vi "Set All Elements.vi"(8 "error in":errorcluster, 10 "Channel Node":refnum<k20>, 11 "Channel Ref in":refnum<data-value>) -> (0 "error out":errorcluster, 3 "Channel Ref out":refnum<data-value>)   [LabVIEW 2024, in "Config File Parser.lvlib" / "Channel.lvclass"]
uses:
  Channel.lvclass
  Channel.lvclass/Channel.ctl
  <vilib>/xml/Close Reference(Node).vi
  Config File Parser.lvlib
  <resource>/objmgr/DOMUserDefRef.rc
  <vilib>/xml/NI_XML.lvlib
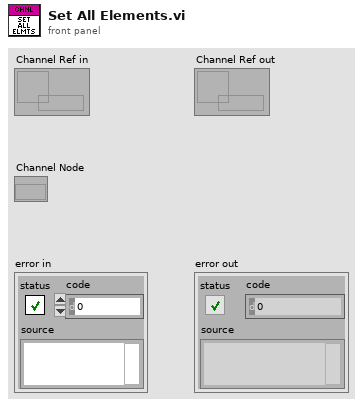
[diagram p1: front panel]
types:
  T1 = cluster{"Key":string, "IsError":bool, "Code":u32, "Message":string}[]
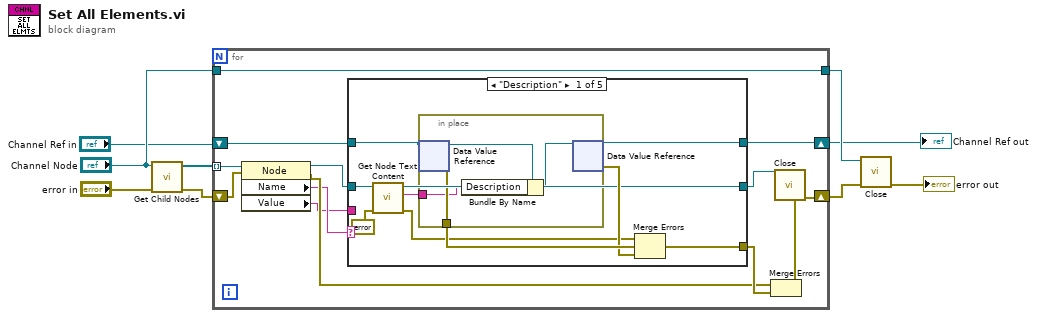
[diagram p0: block diagram]
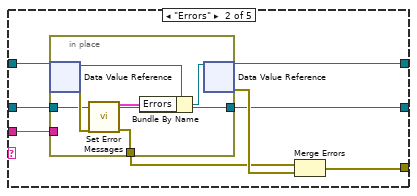
[diagram p2: hidden frame]
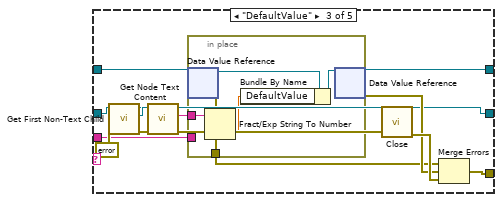
[diagram p3: hidden frame]
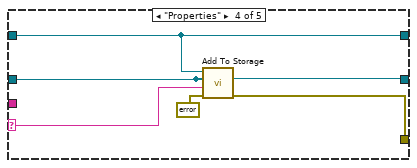
[diagram p4: hidden frame]
diagram:
  n1 = call "Get Child Nodes.vi"("error in"="error in", "Node"="Channel Node") -> ("error out"=w8:errorcluster, "Child Nodes"=w5:refnum<k20>[])  [unwired: 8 in]
  n2 = for {
    tunnel: w5 -> [w17] mode=indexing
    shift-right: [w21] -> w7
    shift-left: w8 -> [w22]
    tunnel: [w13] -> w4
    tunnel: "Channel Node" -> [w13]
    shift-right: [w10] -> w1
    shift-left: "Channel Ref in" -> [w11]
    n3 = property on="Property Node" class="Node"(reference=w17, error in=w22) -> (reference out=w15:refnum<k20>, error out=w19:errorcluster, "Name"=w16:string, "Value"=w14:string)
    n4 = case shown="\"Description\"" w16 {
      selector: w16 -> [_ _ _ w73 _]
      tunnel: w15 -> [w27 w38 w55 w72 w76]
      tunnel: w14 -> [_ w40 w57 _ _]
      tunnel: [w26 w37 w51 w72 w76] -> w12
      tunnel: w11 -> [w29 w41 w58 w71 w77]
      tunnel: [w30 w44 w60 w75 _] -> w20
      tunnel: [w28 w39 w56 w71 w77] -> w10
      frame "Description" {
        n5 = call <vilib>:"Get Node Text Content.vi"("error in (no error)"=errorcluster {"status"=FALSE, "code"=0, "source"=""}, "node in"=w27) -> ("error out"=w23:errorcluster, "node text"=w24:string, "node out"=w26:refnum<k20>)  [unwired: 7 in]
        n6 = in-place "In Place Element Structure" {
          in-place-border: [w36] -> w32
          in-place-border: w24 -> [w33]
          n7 = in-place-dvr #1(w29) -> (w35:refnum<class "Channel.lvclass">, w36:errorcluster)
          n8 = Bundle By Name(cluster=w35, "Description"=w33) -> (w34:refnum<class "Channel.lvclass">)
          n9 = in-place-dvr #1(w34) -> (w28:refnum<data-value>, w31:errorcluster)
        }
        n10 = Merge Errors(w23, w32, w31) -> (w30:errorcluster)
      }
      frame "Errors" {
        n11 = in-place "In Place Element Structure" {
          in-place-border: w40 -> [_]
          in-place-border: w38 -> [w45]
          in-place-border: [w49] -> w42
          in-place-border: [w45] -> w37
          n12 = in-place-dvr #2(w41) -> (w48:refnum<class "Channel.lvclass">, w50:errorcluster)
          n13 = call "Set Error Messages.vi"("error in"=w50, "Errors Node"=w45) -> ("error out"=w49:errorcluster, "Errors"=w46:T1)  [unwired: 8 in]
          n14 = Bundle By Name(cluster=w48, "Errors"=w46) -> (w47:refnum<class "Channel.lvclass">)
          n15 = in-place-dvr #2(w47) -> (w39:refnum<data-value>, w43:errorcluster)
        }
        n16 = Merge Errors(w42, w43) -> (w44:errorcluster)
      }
      frame "DefaultValue" {
        n17 = call <vilib>:"Get First Non-Text Child.vi"("error in (no error)"=errorcluster {"status"=FALSE, "code"=0, "source"=""}, "node in"=w55) -> ("error out"=w64:errorcluster, "child node"=w54:refnum<k20>, "node out"=w51:refnum<k20>)  [unwired: 6 in, 1 out]
        n18 = call <vilib>:"Get Node Text Content.vi"("error in (no error)"=w64, "node in"=w54) -> ("error out"=w63:errorcluster, "node text"=w53:string, "node out"=w52:refnum<k20>)  [unwired: 7 in]
        n19 = in-place "In Place Element Structure" {
          in-place-border: w57 -> [_]
          in-place-border: [w70] -> w59
          in-place-border: w53 -> [w67]
          n20 = in-place-dvr #3(w58) -> (w69:refnum<class "Channel.lvclass">, w70:errorcluster)
          n21 = Fract/Exp String To Number(string=w67) -> (number=w66:dbl)  [unwired: 3 in, 1 out]
          n22 = Bundle By Name(cluster=w69, "DefaultValue"=w66) -> (w68:refnum<class "Channel.lvclass">)
          n23 = in-place-dvr #3(w68) -> (w56:refnum<data-value>, w61:errorcluster)
        }
        n24 = call-poly <vilib>:"Close.vi"("error in (no error)"=w63, "node"=w52) -> ("error out"=w62:errorcluster)  [unwired: 7 in]
        n25 = Merge Errors(w59, w61, w62) -> (w60:errorcluster)
      }
      frame "Properties" {
        n26 = call "Add To Storage.vi"("error in"=errorcluster {"status"=FALSE, "code"=0, "source"=""}, "Item Name"=w73, "Item node"=w72, "Item Ref in"=w71) -> ("error out"=w75:errorcluster)  [unwired: 6 in, 1 out]
      }
      frame "-1", Default {
      }
    }
    n27 = Merge Errors(w19, w20) -> (w18:errorcluster)
    n28 = call-poly <vilib>:"Close.vi"("error in (no error)"=w18, "node"=w12) -> ("error out"=w21:errorcluster)  [unwired: 7 in]
  }
  "Channel Ref out" <- w1
  n29 = call-poly <vilib>:"Close.vi"("error in (no error)"=w7, "node"=w4) -> ("error out"=→"error out":errorcluster)  [unwired: 7 in]
